vi "Serial.vi"(6 "Close":bool, 8 "error in (no error)":errorcluster, 9 "Clear Log":bool, 10 "write buffer":string="UA[3]\r\n", 11 "VISA resource name":refnum<visa-resource-name>="COM6") -> (0 "error out":errorcluster, 2 "read buffer":string)   [LabVIEW 2017]
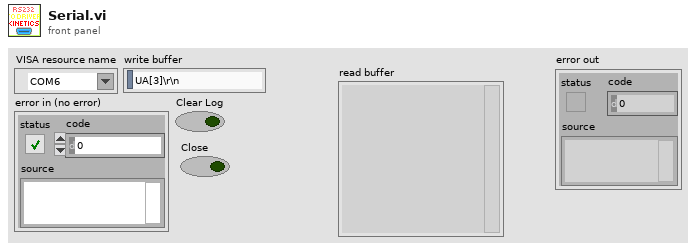
[diagram p1: front panel]
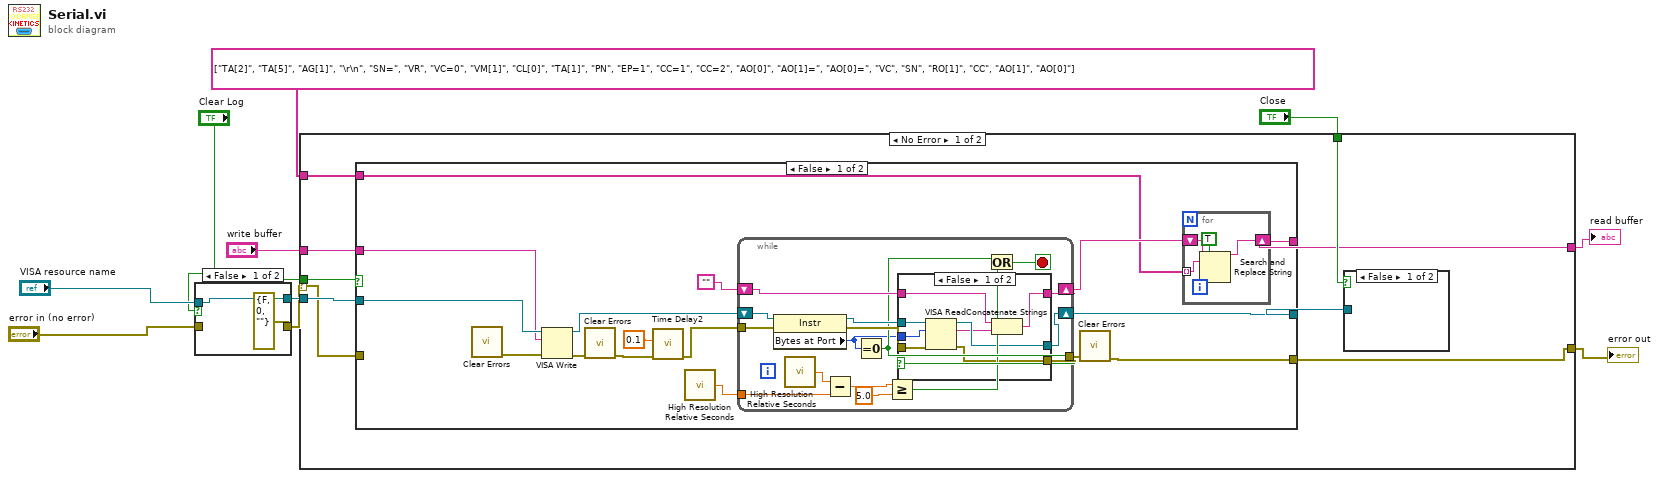
[diagram p0: block diagram]
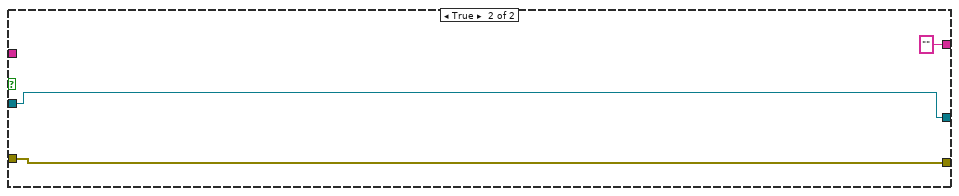
[diagram p3: hidden frame]
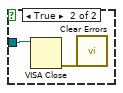
[diagram p4: hidden frame]
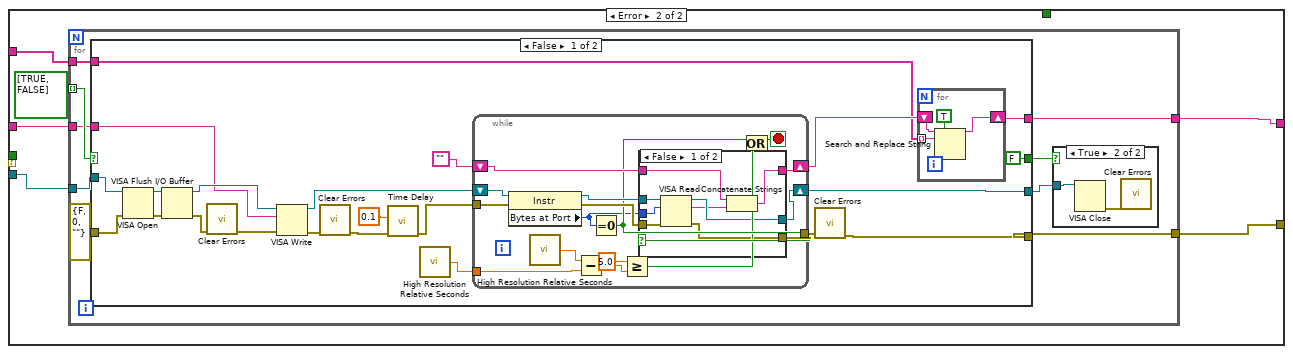
[diagram p5: hidden frame]
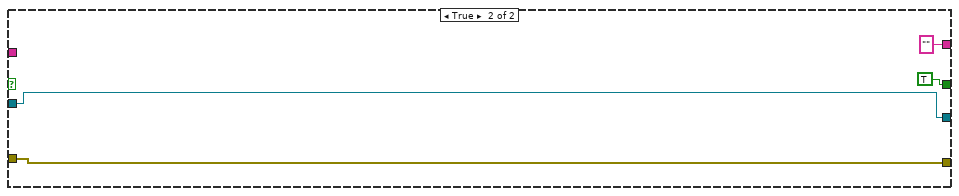
[diagram p7: hidden frame]
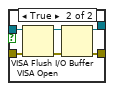
[diagram p9: hidden frame]
diagram:
  n1 = case shown="False" "Clear Log" {
    tunnel: "error in (no error)" -> [_ w18]
    tunnel: "VISA resource name" -> [w12 w17]
    tunnel: [w12 w14] -> w8
    tunnel: [errorcluster {"status"=FALSE, "code"=0, "source"=""} ("error out") w13] -> w6
    frame False {
    }
    frame True {
      n2 = VISA Open(error in (no error)=w18, VISA resource name=w17) -> (VISA resource name=w15:refnum<visa-resource-name>, error out=w16:errorcluster)  [unwired: 3 in]
      n3 = VISA Flush I/O Buffer(VISA resource name=w15, error in (no error)=w16) -> (VISA resource name out=w14:refnum<visa-resource-name>, error out=w13:errorcluster)  [unwired: 1 in]
    }
  }
  n4 = case shown="No Error" w6 {
    selector: w6 -> [w22 _]
    tunnel: w8 -> [w26 w85]
    tunnel: "Clear Log" -> [w19 _]
    tunnel: "Close" -> [w25 _]
    tunnel: [w24 w84] -> w4
    tunnel: [w23 w83] -> w3
    tunnel: "write buffer" -> [w21 w81]
    tunnel: string[] ["TA[2]", "TA[5]", "AG[1]", "\r\n", "SN=", "VR", "VC=0", "VM[1]", "CL[0]", "TA[1]", "PN", "EP=1", "CC=1", "CC=2", "AO[0]", "AO[1]=", "AO[0]=", "VC", "SN", "RO[1]", "CC", "AO[1]", "AO[0]"] -> [w20 w80]
    frame No Error {
      n5 = case shown="False" w19 {
        tunnel: [w42 w75] -> w23
        tunnel: [w41 w76] -> w27
        tunnel: [w32 ""] -> w24
        tunnel: w26 -> [w30 w76]
        tunnel: w22 -> [_ w75]
        tunnel: w21 -> [w29 _]
        tunnel: w20 -> [w28 _]
        frame False {
          n6 = call <vilib>:"Clear Errors.vi"() -> ("error out"=w37:errorcluster)  [unwired: 6 in, 1 out]
          n7 = VISA Write(VISA resource name=w30, write buffer=w29, error in (no error)=w37) -> (VISA resource name out=w36:refnum<visa-resource-name>, error out=w40:errorcluster)  [unwired: 1 out]
          n8 = call <vilib>:"Clear Errors.vi"("error in (no error)"=w40) -> ("error out"=w39:errorcluster)  [unwired: 5 in, 1 out]
          n9 = call "Time Delay2"("error in (no error)"=w39, "Delay Time (s)"=0.1) -> ("error out"=w35:errorcluster)  [unwired: 9 in]
          n10 = call <vilib>:"High Resolution Relative Seconds.vi"() -> ("relative seconds"=w31:dbl)
          n11 = while {
            shift-right: [w62] -> w41
            shift-left: w36 -> [w61]
            tunnel: [w63] -> w43
            tunnel: w35 -> [w59]
            shift-right: [w57] -> w33
            shift-left: "" -> [w58]
            tunnel: w31 -> [w51]
            stop <- w53 stop-if-true
            n12 = property class="Instr"(reference=w61, error in=w59) -> (reference out=w60:refnum<visa-resource-name>, error out=w56:errorcluster, "Bytes at Port"=w54:u32)
            n13 = call <vilib>:"High Resolution Relative Seconds.vi"() -> ("relative seconds"=w52:dbl)
            n14 = Subtract(x=w52, y=w51) -> (x-y=w50:dbl)
            n15 = Equal To 0?(x=w54) -> (x = 0?=w55:bool)
            n16 = Greater Or Equal?(x=w50, y=5.0 ("x")) -> (x >= y?=w48:bool)
            n17 = case shown="False" w55 {
              tunnel: [w71 w72] -> w63
              tunnel: [w70 w73] -> w62
              tunnel: w60 -> [w69 w73]
              tunnel: w58 -> [w67 w74]
              tunnel: [w66 w74] -> w57
              tunnel: w56 -> [w65 w72]
              tunnel: w54 -> [w64 _]
              frame False {
                n18 = VISA Read(VISA resource name=w69, byte count=w64, error in (no error)=w65) -> (VISA resource name out=w70:refnum<visa-resource-name>, read buffer=w68:string, error out=w71:errorcluster)  [unwired: 1 out]
                n19 = Concatenate Strings(w67, w68) -> (w66:string)
              }
              frame True {
              }
            }
            n20 = Or(x=w55, y=w48) -> (x .or. y?=w53:bool)
          }
          n21 = call <vilib>:"Clear Errors.vi"("error in (no error)"=w43) -> ("error out"=w42:errorcluster)  [unwired: 5 in, 1 out]
          n22 = for {
            shift-right: [w45] -> w32
            shift-left: w33 -> [w46]
            tunnel: w28 -> [w44] mode=indexing
            n23 = Search and Replace String(replace all?=TRUE ("replace all? (F)"), input string=w46, search string=w44) -> (result string=w45:string)  [unwired: 5 in, 3 out]
          }
        }
        frame True {
        }
      }
      n24 = case shown="False" w25 {
        tunnel: w27 -> [_ w78]
        frame False {
        }
        frame True {
          n25 = VISA Close(VISA resource name=w78) -> (error out=w79:errorcluster)  [unwired: 1 in]
          n26 = call <vilib>:"Clear Errors.vi"("error in (no error)"=w79) -> ()  [unwired: 5 in, 2 out]
        }
      }
    }
    frame Error {
      n27 = for {
        tunnel: w85 -> [w93]
        tunnel: [w92] -> w84
        tunnel: [w91] -> w83
        tunnel: bool[] [TRUE, FALSE] -> [w89] mode=indexing
        tunnel: w81 -> [w87]
        tunnel: w80 -> [w86]
        n28 = case shown="False" w89 {
          tunnel: [w115 w149] -> w91
          tunnel: [w114 w150] -> w94
          tunnel: [w105 ""] -> w92
          tunnel: w93 -> [w102 w150]
          tunnel: errorcluster {"status"=FALSE, "code"=0, "source"=""} ("error out") -> [w101 w149]
          tunnel: [FALSE TRUE] -> w88
          tunnel: w87 -> [w96 _]
          tunnel: w86 -> [w95 _]
          frame False {
            n29 = VISA Open(error in (no error)=w101, VISA resource name=w102) -> (VISA resource name=w100:refnum<visa-resource-name>, error out=w103:errorcluster)  [unwired: 3 in]
            n30 = VISA Flush I/O Buffer(VISA resource name=w100, error in (no error)=w103) -> (VISA resource name out=w99:refnum<visa-resource-name>, error out=w98:errorcluster)  [unwired: 1 in]
            n31 = call <vilib>:"Clear Errors.vi"("error in (no error)"=w98) -> ("error out"=w110:errorcluster)  [unwired: 5 in, 1 out]
            n32 = VISA Write(VISA resource name=w99, write buffer=w96, error in (no error)=w110) -> (VISA resource name out=w109:refnum<visa-resource-name>, error out=w113:errorcluster)  [unwired: 1 out]
            n33 = call <vilib>:"Clear Errors.vi"("error in (no error)"=w113) -> ("error out"=w112:errorcluster)  [unwired: 5 in, 1 out]
            n34 = call "Time Delay"("error in (no error)"=w112, "Delay Time (s)"=0.1) -> ("error out"=w108:errorcluster)  [unwired: 9 in]
            n35 = call <vilib>:"High Resolution Relative Seconds.vi"() -> ("relative seconds"=w104:dbl)
            n36 = while {
              shift-right: [w135] -> w114
              shift-left: w109 -> [w134]
              tunnel: [w136] -> w116
              tunnel: w108 -> [w132]
              shift-right: [w130] -> w106
              shift-left: "" -> [w131]
              tunnel: w104 -> [w124]
              stop <- w126 stop-if-true
              n37 = property class="Instr"(reference=w134, error in=w132) -> (reference out=w133:refnum<visa-resource-name>, error out=w129:errorcluster, "Bytes at Port"=w127:u32)
              n38 = call <vilib>:"High Resolution Relative Seconds.vi"() -> ("relative seconds"=w125:dbl)
              n39 = Subtract(x=w125, y=w124) -> (x-y=w123:dbl)
              n40 = Equal To 0?(x=w127) -> (x = 0?=w128:bool)
              n41 = Greater Or Equal?(x=5.0, y=w123) -> (x >= y?=w121:bool)
              n42 = case shown="False" w128 {
                tunnel: [w144 w145] -> w136
                tunnel: [w143 w146] -> w135
                tunnel: w133 -> [w142 w146]
                tunnel: w131 -> [w140 w147]
                tunnel: [w139 w147] -> w130
                tunnel: w129 -> [w138 w145]
                tunnel: w127 -> [w137 _]
                frame False {
                  n43 = VISA Read(VISA resource name=w142, byte count=w137, error in (no error)=w138) -> (VISA resource name out=w143:refnum<visa-resource-name>, read buffer=w141:string, error out=w144:errorcluster)  [unwired: 1 out]
                  n44 = Concatenate Strings(w140, w141) -> (w139:string)
                }
                frame True {
                }
              }
              n45 = Or(x=w128, y=w121) -> (x .or. y?=w126:bool)
            }
            n46 = call <vilib>:"Clear Errors.vi"("error in (no error)"=w116) -> ("error out"=w115:errorcluster)  [unwired: 5 in, 1 out]
            n47 = for {
              tunnel: w95 -> [w119] mode=indexing
              shift-right: [w117] -> w105
              shift-left: w106 -> [w118]
              n48 = Search and Replace String(replace all?=TRUE ("replace all? (F)"), input string=w118, search string=w119) -> (result string=w117:string)  [unwired: 5 in, 3 out]
            }
          }
          frame True {
          }
        }
        n49 = case shown="True" w88 {
          tunnel: w94 -> [_ w152]
          frame False {
          }
          frame True {
            n50 = VISA Close(VISA resource name=w152) -> (error out=w153:errorcluster)  [unwired: 1 in]
            n51 = call <vilib>:"Clear Errors.vi"("error in (no error)"=w153) -> ()  [unwired: 5 in, 2 out]
          }
        }
      }
    }
  }
  "read buffer" <- w4
  "error out" <- w3
